vi "Add Objects.vi"(8 "error in":errorcluster, 10 "elements":refnum<class>[](array[class]), 11 "Buffer in":refnum<data-value>) -> (0 "error out":errorcluster, 2 "overflow":refnum<class>[](array[class]), 3 "Buffer":refnum<data-value>)   [LabVIEW 2013, in "CircularBuffer.lvlib" / "ObjectBuffer.lvclass"]
doc: "This VI allows to input an array into the buffer. The location in the buffer is updated automatically.\n\nIf the input array is larger than the buffer then just take last elements of the input array and save them in the buffer. Also give a warning that this happened."
uses:
  ObjectBuffer.lvclass
  VariantBuffer/VariantBuffer.lvclass
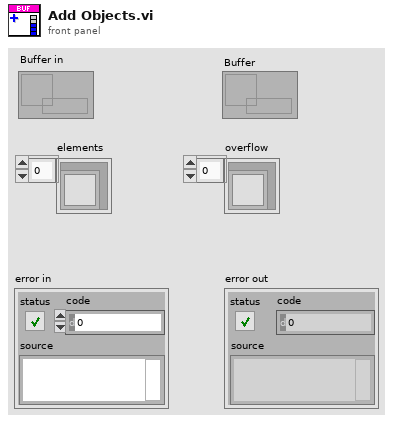
[diagram p1: front panel]
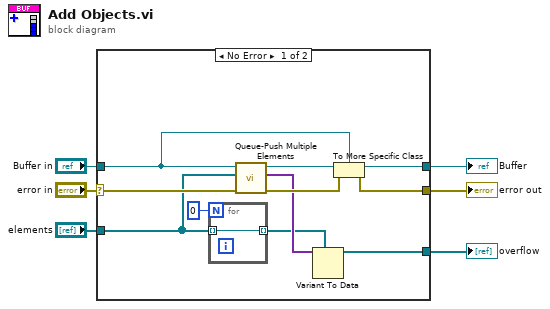
[diagram p0: block diagram]
diagram:
  n1 = case shown="No Error" "error in" {
    selector: "error in" -> [w14 w20]
    tunnel: "Buffer in" -> [w15 w19]
    tunnel: [w12 w19] -> w5
    tunnel: [w13 w20] -> w4
    tunnel: "elements" -> [w10 _]
    tunnel: [w7 _] -> w1
    frame No Error {
      n2 = for {
        N: 0 -> [_]
        tunnel: w10 -> [w18] mode=indexing
        tunnel: [w18] -> w9 mode=indexing
      }
      n3 = call "Queue-Push Multiple Elements.vi"("error in"=w14, "elements"=w10, "Buffer in"=w15) -> ("error out"=w16:errorcluster, "overflow"=w11:variant[], "Buffer"=w17:refnum<data-value>)  [unwired: 6 in]
      n4 = Variant To Data(type=w9, Variant=w11) -> (data=w7:refnum<class>[])  [unwired: 1 in, 1 out]
      n5 = To More Specific Class(target class=w15, reference=w17, error in=w16) -> (specific class reference=w12:refnum<data-value>, error out=w13:errorcluster)
    }
    frame Error {
    }
  }
  "error out" <- w4
  "Buffer" <- w5
  "overflow" <- w1
